vi "sv_Check Custom IMD Settings.vi"(5 "frequency range":T1 {"stop frequency" format="%.2f"; "start frequency" format="%.2f"}, 7 "RBW":dbl format="%.2f", 11 "error in (no error)":errorcluster, 12 "custom IMD settings":T3={"IMD type"=enum."SMPTE/DIN", "low-frequency tone"=-1.0, "high-frequency tone"=-1.0, "amplitude ratio"=-1.0, "maximum order"=-1} {"amplitude ratio" format="%.2f"; "high-frequency tone" format="%.2f"; "low-frequency tone" format="%.2f"}, 13 "IMD standard":T2(ring)=enum."Custom") -> (14 "dup custom IMD settings":T3 {"amplitude ratio" format="%.2f"; "high-frequency tone" format="%.2f"; "low-frequency tone" format="%.2f"}, 15 "error out":errorcluster)   [LabVIEW 2017, in "SoundVib_Distortion.lvlib"]
uses:
  <vilib>/addons/Sound and Vibration/svt_Distortion/SoundVib_Distortion.lvlib
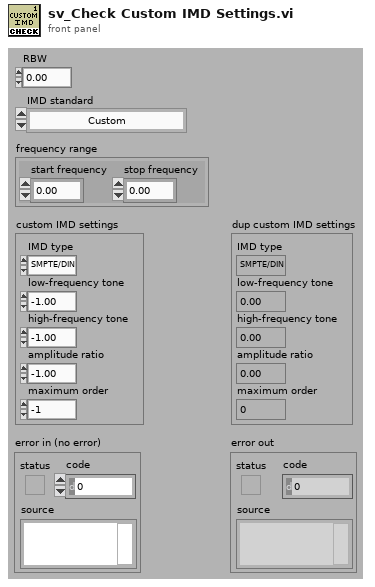
[diagram p1: front panel]
types:
  T1 = cluster{"start frequency":dbl, "stop frequency":dbl}
  T2 = enum16{"SMPTE (60 Hz, 7000 Hz, 4:1)", "DIN (250 Hz, 8000 Hz, 4:1)", "CCIF (11 kHz, 12 kHz, 1:1)", "CCIF (19 kHz, 20 kHz, 1:1)", "Custom"}
  T3 = cluster{"IMD type":enum16{"SMPTE/DIN", "CCIF/Twin-Tone"}, "low-frequency tone":dbl, "high-frequency tone":dbl, "amplitude ratio":dbl, "maximum order":i32}
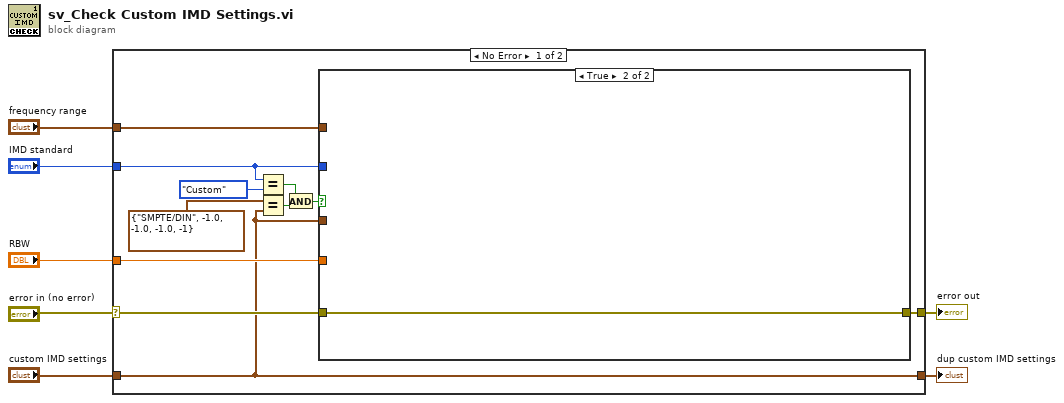
[diagram p0: block diagram]
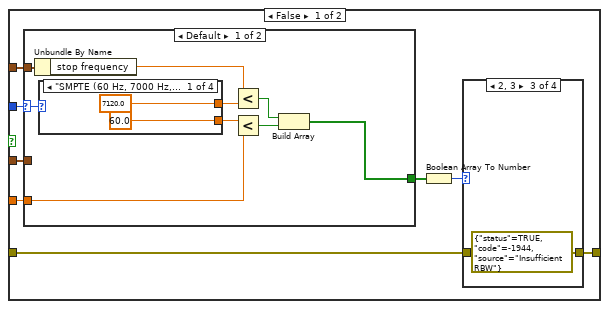
[diagram p2: hidden frame]
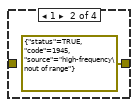
[diagram p4: hidden frame]
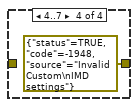
[diagram p5: hidden frame]
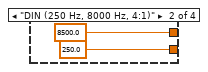
[diagram p6: hidden frame]
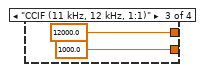
[diagram p7: hidden frame]
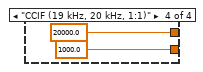
[diagram p8: hidden frame]
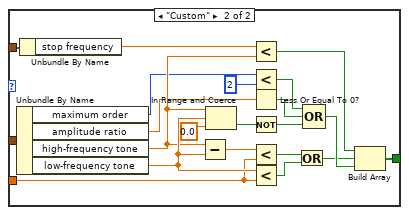
[diagram p9: hidden frame]
diagram:
  n1 = case shown="No Error" "error in (no error)" {
    selector: "error in (no error)" -> [w16 w71]
    tunnel: "custom IMD settings" -> [w13 w70]
    tunnel: "RBW" -> [w18 _]
    tunnel: [w15 w71] -> w4
    tunnel: [w13 w70] -> w5
    tunnel: "IMD standard" -> [w14 _]
    tunnel: "frequency range" -> [w17 _]
    frame No Error {
      n2 = Equal?(x=w14, y=T2."Custom") -> (x = y?=w9:bool)
      n3 = Equal?(x=T3 {"IMD type"=enum."SMPTE/DIN", "low-frequency tone"=-1.0, "high-frequency tone"=-1.0, "amplitude ratio"=-1.0, "maximum order"=-1}, y=w13) -> (x = y?=w10:bool)
      n4 = And(x=w9, y=w10) -> (x .and. y?=w8:bool)
      n5 = case shown="True" w8 {
        tunnel: w18 -> [w26 _]
        tunnel: w17 -> [w25 _]
        tunnel: w16 -> [w23 w69]
        tunnel: [w21 w69] -> w15
        tunnel: w14 -> [w20 _]
        tunnel: w13 -> [w19 _]
        frame False {
          n6 = case shown="Default" w20 {
            selector: w20 -> [w39 _]
            tunnel: w26 -> [w38 w51]
            tunnel: w19 -> [_ w67]
            tunnel: w25 -> [w37 w59]
            tunnel: [w31 w50] -> w24
            frame Default {
              n7 = Unbundle By Name(w37) -> ("stop frequency"=w36:dbl)
              n8 = case shown="\"SMPTE (60 Hz, 7000 Hz, 4:1)\", Default" w39 {
                tunnel: [7120.0 8500.0 12000.0 20000.0] -> w35
                tunnel: [60.0 250.0 1000.0 1000.0] -> w34
                frame "SMPTE (60 Hz, 7000 Hz, 4:1)", Default {
                }
                frame "DIN (250 Hz, 8000 Hz, 4:1)" {
                }
                frame "CCIF (11 kHz, 12 kHz, 1:1)" {
                }
                frame "CCIF (19 kHz, 20 kHz, 1:1)" {
                }
              }
              n9 = Less?(x=w36, y=w35) -> (x < y?=w32:bool)
              n10 = Less?(x=w34, y=w38) -> (x < y?=w33:bool)
              n11 = Build Array(w32, w33) -> (w31:bool[])
            }
            frame "Custom" {
              n12 = Unbundle By Name(w67) -> ("maximum order"=w55:i32, "amplitude ratio"=w54:dbl, "high-frequency tone"=w57:dbl, "low-frequency tone"=w68:dbl)
              n13 = Unbundle By Name(w59) -> ("stop frequency"=w58:dbl)
              n14 = Subtract(x=w57, y=w68) -> (x-y=w66:dbl)
              n15 = In Range and Coerce(upper limit=w57, x=w68, lower limit=0.0 ("upper limit")) -> (In Range?=w62:bool)  [unwired: 1 out]
              n16 = Less?(x=w58, y=w57) -> (x < y?=w56:bool)
              n17 = Less?(x=w55, y=2) -> (x < y?=w53:bool)
              n18 = Less Or Equal To 0?(x=w54) -> (x <= 0?=w52:bool)
              n19 = Not(x=w62) -> (.not. x?=w61:bool)
              n20 = Less?(x=w66, y=w51) -> (x < y?=w64:bool)
              n21 = Less?(x=w68, y=w51) -> (x < y?=w63:bool)
              n22 = Or(x=w64, y=w63) -> (x .or. y?=w48:bool)
              n23 = Compound Arithmetic op=OR(w53, w52, w61) -> (w49:bool)
              n24 = Build Array(w56, w48, w49) -> (w50:bool[])
            }
          }
          n25 = Boolean Array To Number(Boolean array=w24) -> (number=w22:u32)
          n26 = case shown="2, 3" w22 {
            tunnel: w23 -> [w27 _ _ _]
            tunnel: [w27 errorcluster {"status"=TRUE, "code"=1945, "source"="high-frequency\nout of range"} ("error IO") errorcluster {"status"=TRUE, "code"=-1944, "source"="Insufficient RBW"} ("error IO") errorcluster {"status"=TRUE, "code"=-1948, "source"="Invalid Custom\nIMD settings"} ("error IO")] -> w21
            frame 0, Default {
            }
            frame 1 {
            }
            frame 2, 3 {
            }
            frame 4..7 {
            }
          }
        }
        frame True {
        }
      }
    }
    frame Error {
    }
  }
  "dup custom IMD settings" <- w5
  "error out" <- w4
